vi "Start.vi"(5 "Cluster":string, 7 "System":string, 8 "error in (no error)":errorcluster, 9 "DiscoveryPort":u16, 10 "Discovery Address":string, 11 "TelemetryDebug in":refnum<class "TelemetryDebug.lvclass">) -> (0 "error out":errorcluster, 3 "TelemetryDebug out":refnum<class "TelemetryDebug.lvclass">)   [LabVIEW 2020, in "VectoTools.lvlib" / "TelemetryDebug.lvclass"]
uses:
  TelemetryDebug.lvclass
  Vecto/NodeDiscovery/NodeDiscovery.lvclass
  Vecto/Node Config/Node Config.lvclass
  Vecto/Node Config/Node Info.ctl
  Vecto/SequenceCountService/SequenceCountService.lvclass
  Vecto/Node Config/Discovery Info.ctl
  Vecto/RemoteDataService/RemoteDataService.lvclass
  Vecto/ChannelService/ChannelService.lvclass
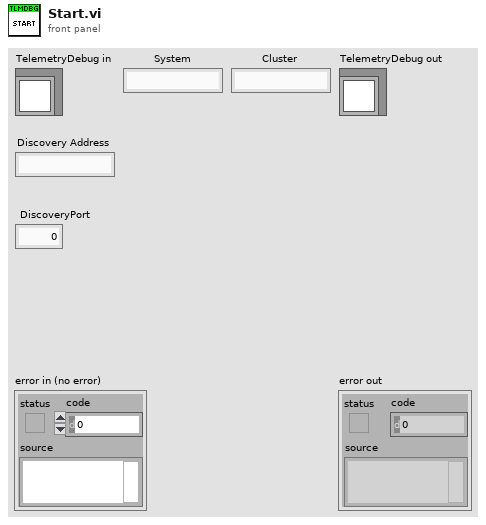
[diagram p1: front panel]
types:
  T1 = typedef "Vecto.lvlib/Node Config.lvclass/Discovery Info.ctl" = cluster{"Address":string, "Port":u16, "Interval S":dbl, "Bind Address":string}
  T2 = typedef "Vecto.lvlib/Node Config.lvclass/Node Info.ctl" = cluster{"System":string, "Cluster":string, "Name":string, "ID":u32}
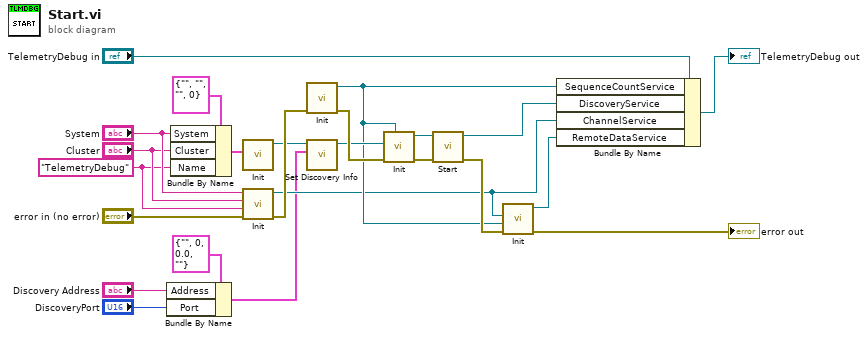
[diagram p0: block diagram]
diagram:
  w8 = "TelemetryDebug" ("Name")
  n1 = Bundle By Name(cluster=T1 {"Address"="", "Port"=0, "Interval S"=0.0, "Bind Address"=""} ("Discovery Info"), "Address"="Discovery Address", "Port"="DiscoveryPort") -> (w1:T1)
  n2 = Bundle By Name(cluster=T2 {"System"="", "Cluster"="", "Name"="", "ID"=0} ("Node Info"), "System"="System", "Cluster"="Cluster", "Name"=w8) -> (w20:T2)
  n3 = call "Init.vi"("Node Info"=w20) -> ("Node out"=w19:refnum<class "Node Config.lvclass">)  [unwired: 9 in, 1 out]
  n4 = call "Init.vi"("error in (no error)"="error in (no error)", "Node"=w8, "Cluster"="Cluster", "System"="System") -> ("error out"=w24:errorcluster, "ChannelService out"=w7:refnum<class "ChannelService.lvclass">)  [unwired: 6 in]
  n5 = call "Init.vi"("error in (no error)"=w24) -> ("error out"=w22:errorcluster, "SequenceCountService out"=w11:refnum<class "SequenceCountService.lvclass">)  [unwired: 9 in]
  n6 = call "Set Discovery Info.vi"("Discovery Info"=w1, "Node in"=w19) -> ("Node out"=w17:refnum<class "Node Config.lvclass">)  [unwired: 8 in, 1 out]
  n7 = call "Init.vi"("SequenceCountService"=w11, "error in (no error)"=w22, "Node"=w17) -> ("error out"=w15:errorcluster, "DiscoveryService out"=w16:refnum<class "NodeDiscovery.lvclass">)  [unwired: 7 in]
  n8 = call "Start.vi"("error in (no error)"=w15, "DiscoveryService in"=w16) -> ("error out"=w23:errorcluster, "DiscoveryService out"=w12:refnum<class "NodeDiscovery.lvclass">)  [unwired: 8 in]
  n9 = call "Init.vi"("error in (no error)"=w23, "SequenceCountService"=w11, "ChannelService"=w7) -> ("error out"=→"error out":errorcluster, "RemoteDataService out"=w6:refnum<class "RemoteDataService.lvclass">)  [unwired: 7 in]
  n10 = Bundle By Name(cluster="TelemetryDebug in", "SequenceCountService"=w11, "DiscoveryService"=w12, "ChannelService"=w7, "RemoteDataService"=w6) -> (→"TelemetryDebug out":refnum<class "TelemetryDebug.lvclass">)
